vi "Lezeti_Power_Monitor_05.vi"() -> ()   [LabVIEW 2012]
doc: "This example shows how to use autosetup and acquire a waveform on a single channel."
uses:
  Program Files (x86)/National Instruments/LabVIEW 2012/instr.lib/RIGOL DS1000 Series/Public/Data/Read (Single Waveform).vi
  <vilib>/measure/madcrms.llb/Basic Averaged DC-RMS for 1 Chan.vi
  <vilib>/measure/mascope.llb/Cycle Average and RMS 1 chan.vi
  <vilib>/Utility/file.llb/Write To Spreadsheet File (DBL).vi
  Program Files (x86)/National Instruments/LabVIEW 2012/instr.lib/RIGOL DS1000 Series/RIGOL DS1000 Series.lvlib
  <vilib>/measure/NI_MAPro.lvlib
panel:
  out "Elapsed Time (s)":dbl
  in  "Output File":path
  out "Average Power (Watts)":dbl
  out "Instant Power Waveform":waveform(dbl)(graph)
  in  "Current Channel":u16(ring) items=["Channel 1", "Channel 2", "Channel 3", "Channel 4"]
  in  "Timeout":u32=10000
  out "IRMS":dbl
  out "Current Waveform":waveform(dbl)(graph)
  out "VRMS":dbl
  in  "Voltage Channel":u16(ring) items=["Channel 1", "Channel 2", "Channel 3", "Channel 4"]
  in  "Stop":bool
  in  "Timeout":u32=10000
  out "Voltage Waveform":waveform(dbl)(graph)
  in  "VISA resource name":refnum<visa-resource-name>
  # "For Lezeti Air Conditioning System (Greenpath Tech)\nBy Matsu Thornton\nJuly 2016"
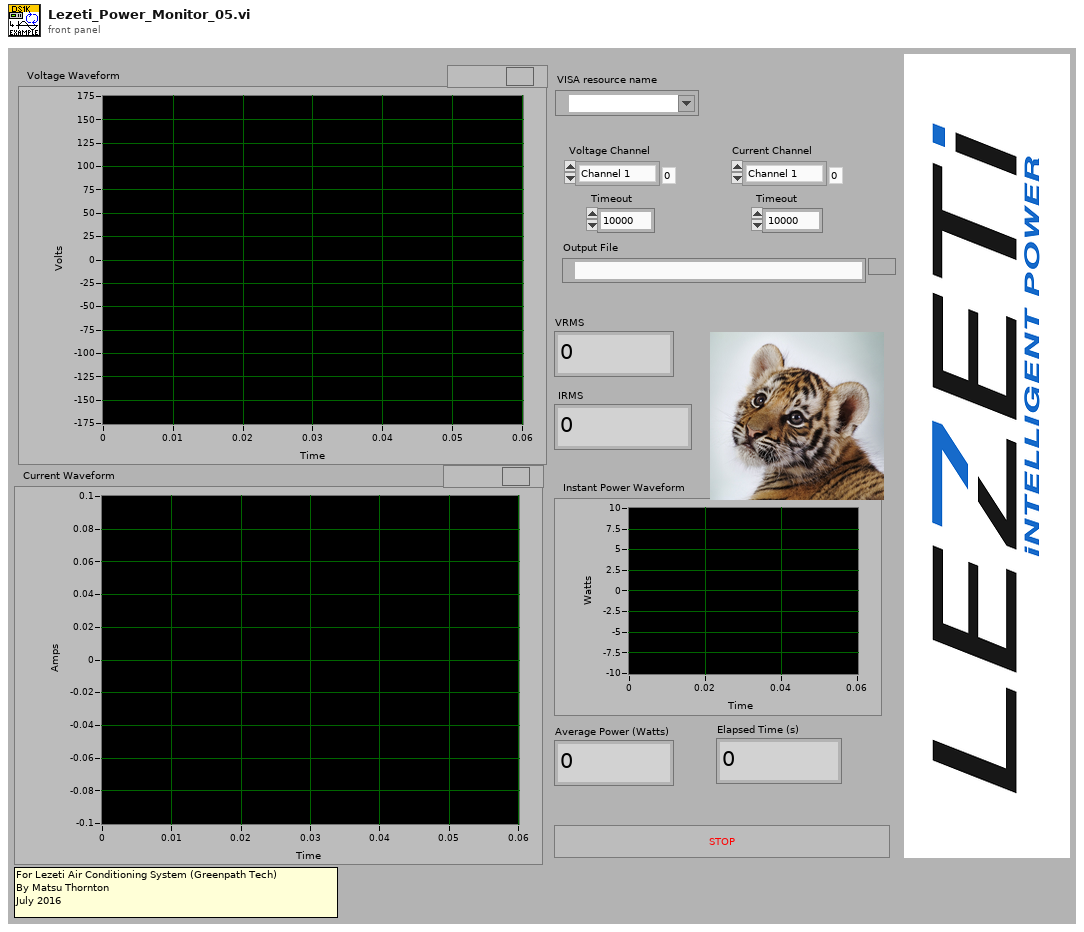
[diagram p1: front panel]
types:
  T1 = typedef "NI_Matrix.lvlib/RealMatrix.ctl" = dbl[][]
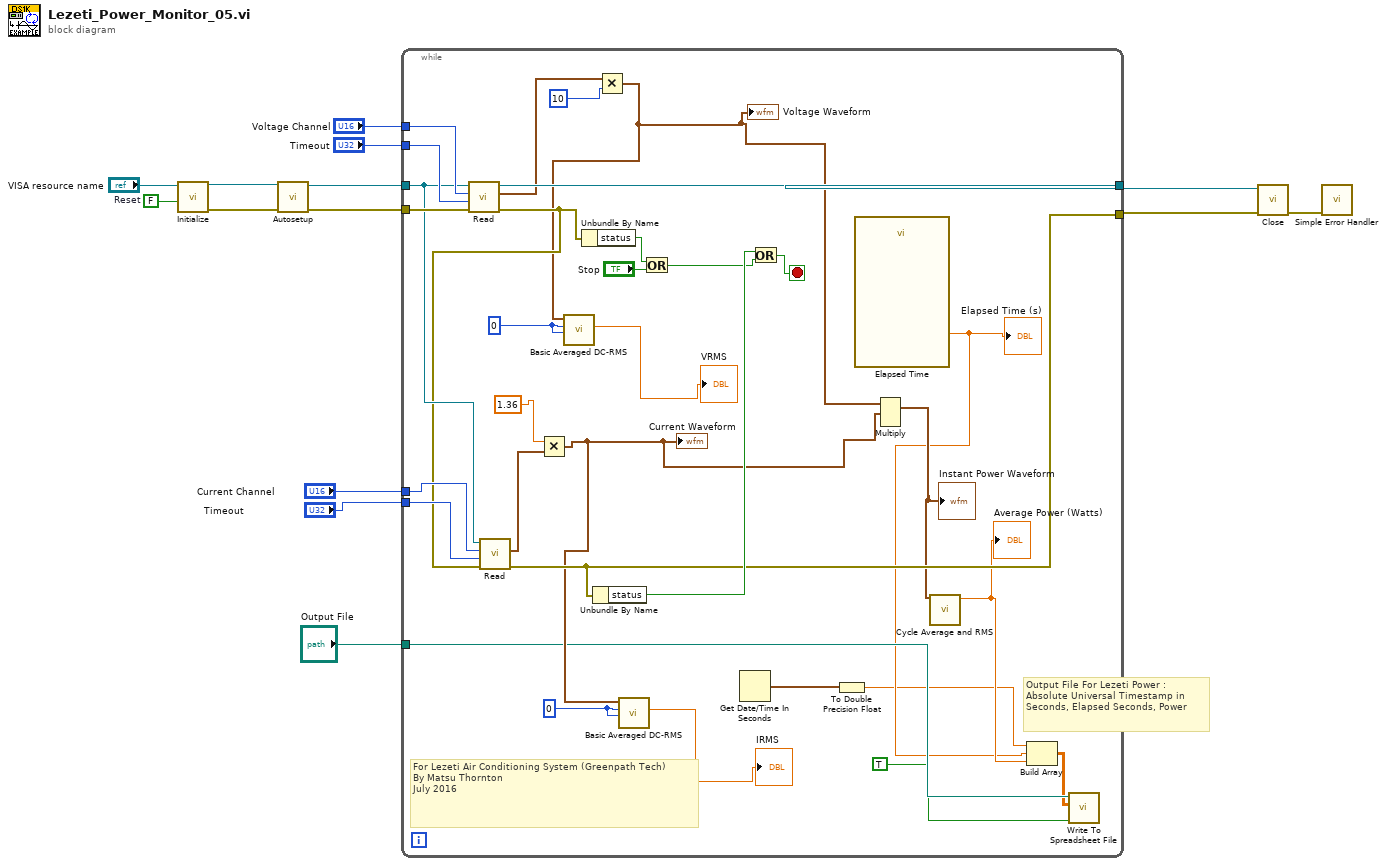
[diagram p0: block diagram]
diagram:
  w5 = FALSE  # Reset
  # "Output File For Lezeti Power :\nAbsolute Universal Timestamp in Seconds, Elapsed Seconds, Power"
  n1 = call "Initialize.vi"("Reset (True)"=w5, "VISA resource name"="VISA resource name") -> ("error out"=w10:errorcluster, "VISA resource name out"=w9:refnum<visa-resource-name>)  [unwired: 2 in, 6 out]
  n2 = call "Autosetup.vi"("error in (no error)"=w10, "VISA resource name"=w9) -> ("error out"=w7:errorcluster, "VISA resource name out"=w8:refnum<visa-resource-name>)  [unwired: 8 out]
  n3 = while {
    tunnel: w8 -> [w35]
    tunnel: w7 -> [w46]
    tunnel: [w45] -> w13
    tunnel: "Timeout" -> [w41]
    tunnel: "Voltage Channel" -> [w42]
    tunnel: "Current Channel" -> [w37]
    tunnel: "Timeout" -> [w36]
    tunnel: [w33] -> w2
    tunnel: "Output File" -> [w21]
    stop <- w23 stop-if-true
    w38 = 0
    w40 = 0
    # "For Lezeti Air Conditioning System (Greenpath Tech)\nBy Matsu Thornton\nJuly 2016"
    n4 = call-poly "Read.vi"("error in (no error)"=w46, "Timeout (10000 ms)"=w41, "Channel (0: Channel 1)"=w42, "VISA resource name"=w35) -> ("error out"=w34:errorcluster, "Waveform Data"=w31:waveform(dbl), "VISA resource name out"=w45:refnum<visa-resource-name>)  [unwired: 5 out]
    n5 = call-poly "Read.vi"("error in (no error)"=w34, "Timeout (10000 ms)"=w36, "Channel (0: Channel 1)"=w37, "VISA resource name"=w35) -> ("error out"=w33:errorcluster, "Waveform Data"=w28:waveform(dbl))  [unwired: 6 out]
    n6 = Multiply(x=1.36, y=w28) -> (x*y=w25:waveform(dbl))
    "Current Waveform" <- w25
    n7 = Unbundle By Name(w34) -> ("status"=w44:bool)
    n8 = Unbundle By Name(w33) -> ("status"=w39:bool)
    n9 = Multiply(x=w31, y=10) -> (x*y=w30:waveform(dbl))
    "Voltage Waveform" <- w30
    n10 = call-poly <vilib>:"Basic Averaged DC-RMS.vi"("window"=w40, "averaging type"=w40, "signal in"=w30) -> ("RMS value"=→"VRMS":dbl)  [unwired: 5 in, 3 out]
    n11 = call-poly <vilib>:"Basic Averaged DC-RMS.vi"("window"=w38, "averaging type"=w38, "signal in"=w25) -> ("RMS value"=→"IRMS":dbl)  [unwired: 5 in, 3 out]
    n12 = Or(x=w44, y="Stop") -> (x .or. y?=w24:bool)
    n13 = Get Date/Time In Seconds() -> (seconds since 1Jan1904=w18:timestamp)
    n14 = Or(x=w39, y=w24) -> (x .or. y?=w23:bool)
    n15 = To Double Precision Float(number=w18) -> (double precision float=w15:dbl)
    n16 = call "Elapsed Time"() -> ("Elapsed Time (s)"=w16:dbl)  [unwired: 12 in, 7 out]
    "Elapsed Time (s)" <- w16
    n17 = Multiply(1:w25, 2:w30) -> (0:w22:waveform(dbl))  [unwired: 1 in, 1 out]
    "Instant Power Waveform" <- w22
    n18 = call-poly <vilib>:"Cycle Average and RMS.vi"("signal in"=w22) -> ("cycle average"=w17:dbl)  [unwired: 7 in, 3 out]
    "Average Power (Watts)" <- w17
    n19 = Build Array(w15, w16, w17) -> (w19:T1)
    n20 = call-poly <vilib>:"Write To Spreadsheet File.vi"("append to file? (new file:F)"=TRUE, "2D data"=w19, "file path (dialog if empty)"=w21) -> ()  [unwired: 5 in, 1 out]
  }
  n21 = call "Close.vi"("error in (no error)"=w2, "VISA resource name"=w13) -> ("error out"=w14:errorcluster)  [unwired: 9 out]
  n22 = call <vilib>:"Simple Error Handler.vi"("error in (no error)"=w14) -> ()  [unwired: 1 in, 8 out]
